vi "m1m3_getEvent_HardpointActuatorInfo.vi"(8 "error in (no error)":errorcluster, 11 "logevent_HardpointActuatorInfo_Ctl":T1) -> (0 "error out":errorcluster, 2 "function return":i32, 3 "logevent_HardpointActuatorInfo_Ctl out":T1)   [LabVIEW 2016, in "SALLV_m1m3.lvlib"]
doc: "int m1m3_shm_getEvent_HardpointActuatorInfoLV(m1m3_logevent_HardpointActuatorInfoLV *logevent_HardpointActuatorInfo_Ctl );"
uses:
  SALLV_m1m3.lvlib
  DataTypes/logevent_HardpointActuatorInfo.ctl
  SALLV_m1m3.so
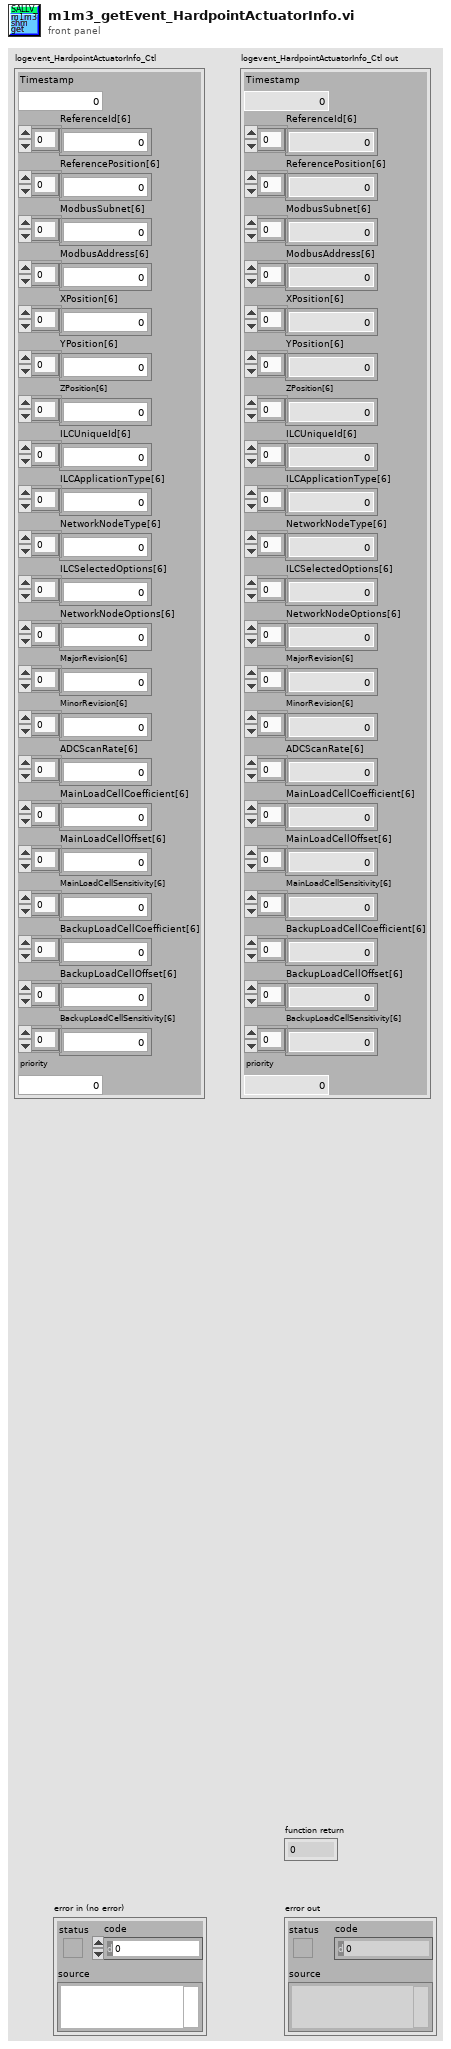
[diagram p1: front panel]
types:
  T1 = typedef "SALLV_m1m3.lvlib/logevent_HardpointActuatorInfo.ctl" = cluster{"Timestamp":dbl, "ReferenceId[6]":i16[], "ReferencePosition[6]":i32[], "ModbusSubnet[6]":i16[], "ModbusAddress[6]":i16[], "XPosition[6]":sgl[], "YPosition[6]":sgl[], "ZPosition[6]":sgl[], "ILCUniqueId[6]":i64[], "ILCApplicationType[6]":i16[], "NetworkNodeType[6]":i16[], "ILCSelectedOptions[6]":i16[], "NetworkNodeOptions[6]":i16[], "MajorRevision[6]":i16[], "MinorRevision[6]":i16[], "ADCScanRate[6]":i16[], "MainLoadCellCoefficient[6]":sgl[], "MainLoadCellOffset[6]":sgl[], "MainLoadCellSensitivity[6]":sgl[], "BackupLoadCellCoefficient[6]":sgl[], "BackupLoadCellOffset[6]":sgl[], "BackupLoadCellSensitivity[6]":sgl[], "priority":i32}
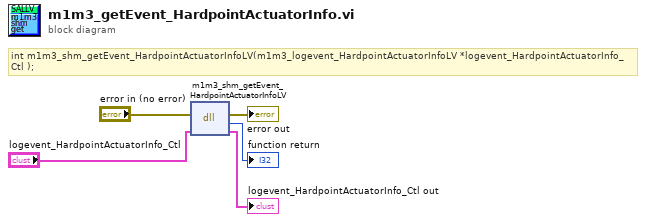
[diagram p0: block diagram]
diagram:
  # "int m1m3_shm_getEvent_HardpointActuatorInfoLV(m1m3_logevent_HardpointActuatorInfoLV *logevent_HardpointActuatorInfo_Ctl );"
  n1 = dll-call lib="opt/CODE/SALLV_m1m3/SALLV_m1m3.*" fn="m1m3_shm_getEvent_HardpointActuatorInfoLV"(error in="error in (no error)", "logevent_HardpointActuatorInfo_Ctl"="logevent_HardpointActuatorInfo_Ctl") -> (error out=→"error out":errorcluster, →"function return":i32, "logevent_HardpointActuatorInfo_Ctl"=→"logevent_HardpointActuatorInfo_Ctl out":T1)  [unwired: 2 in, 1 out]
